vi "setuphardware.vi"(4 "Z Index Terminal":tag="/StimCard/PFI4", 5 "Z Index Enable":bool, 6 "B Input Terminal":tag="/StimCard/PFI11", 7 "Pulses Per Revolution":u32=8000, 8 "error in (no error)":errorcluster, 9 "A Input Terminal":tag="/StimCard/PFI3", 10 "Counter":tag="StimCard/ctr1", 11 "QuadraturePositionDecoder in":refnum<class "QuadraturePositionDecoder.lvclass">) -> (0 "error out":errorcluster, 3 "QuadraturePositionDecoder out":refnum<class "QuadraturePositionDecoder.lvclass">)   [LabVIEW 2014, in "QuadraturePositionDecoder.lvclass"]
uses:
  QuadraturePositionDecoder.lvclass
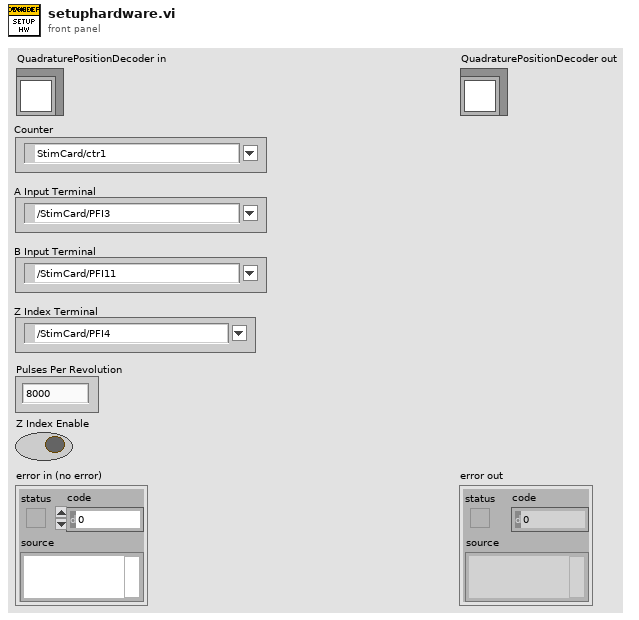
[diagram p1: front panel]
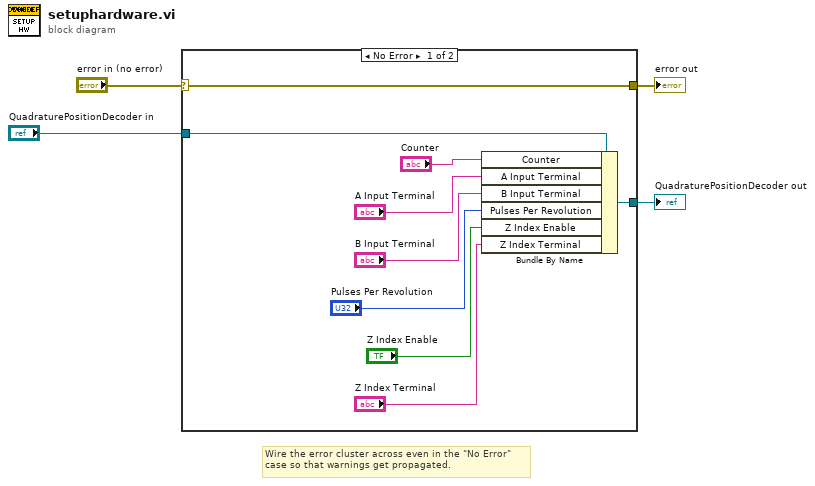
[diagram p0: block diagram]
diagram:
  # "Wire the error cluster across even in the \"No Error\"\ncase so that warnings get propagated."
  n1 = case shown="No Error" "error in (no error)" {
    selector: "error in (no error)" -> [w13 w15]
    tunnel: [w13 w15] -> w3
    tunnel: [w5 w14] -> w1
    tunnel: "QuadraturePositionDecoder in" -> [w12 w14]
    frame No Error {
      n2 = Bundle By Name(cluster=w12, "Counter"="Counter", "A Input Terminal"="A Input Terminal", "B Input Terminal"="B Input Terminal", "Pulses Per Revolution"="Pulses Per Revolution", "Z Index Enable"="Z Index Enable", "Z Index Terminal"="Z Index Terminal") -> (w5:refnum<class "QuadraturePositionDecoder.lvclass">)
    }
    frame Error {
    }
  }
  "error out" <- w3
  "QuadraturePositionDecoder out" <- w1
